vi "Receive Value Change Event.vi"(8 "error in (no error)":errorcluster, 10 "ValueChangeMsg":refnum<class "ValueChangeMsg.lvclass">, 11 "MediatorBusMonitor In":refnum<class "MediatorBusMonitor.lvclass">) -> (0 "error out":errorcluster, 3 "MediatorBusMonitor Out":refnum<class "MediatorBusMonitor.lvclass">)   [LabVIEW 2017, in "Mediator.lvlib" / "MediatorBusMonitor.lvclass"]
doc: "<License>\nCopyright © 2017 Composed Systems, LLC | All rights reserved\nwww.composed.io\n\nAuthor: Ethan Stern <ethan.stern@composed.io>\n\nThis software is provided \"AS IS\" WITHOUT WARRANTIES, either express or implied, AND IS FOR EDUCATIONAL PURPOSES ONLY.\n</License>"
uses:
  MediatorBusMonitor.lvclass
  ActorEvents/IEventAggregator Messages/ValueChangeMsg/ValueChangeMsg.lvclass
  ActorEvents/IEventAggregator Messages/ValueChangeMsg/ValueChangeMsg.lvclass/ValueChangeMsg.ctl
  MediatorBusMonitor.lvclass/MediatorBusMonitor.ctl
  gpm_packages/@cs/lookup-table/Source/LookupTable/LookupTable.lvclass/LookupTable.ctl
  gpm_packages/@cs/lookup-table/Source/LookupTable/Read Table Reference.vi
  gpm_packages/@cs/lookup-table/Source/LookupTable/LookupTable.lvclass
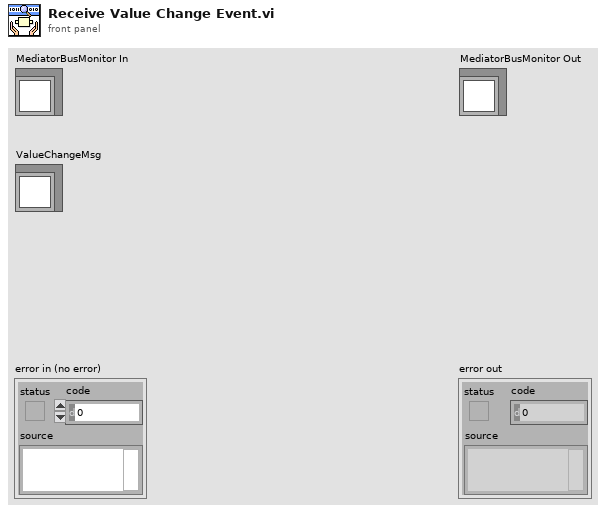
[diagram p1: front panel]
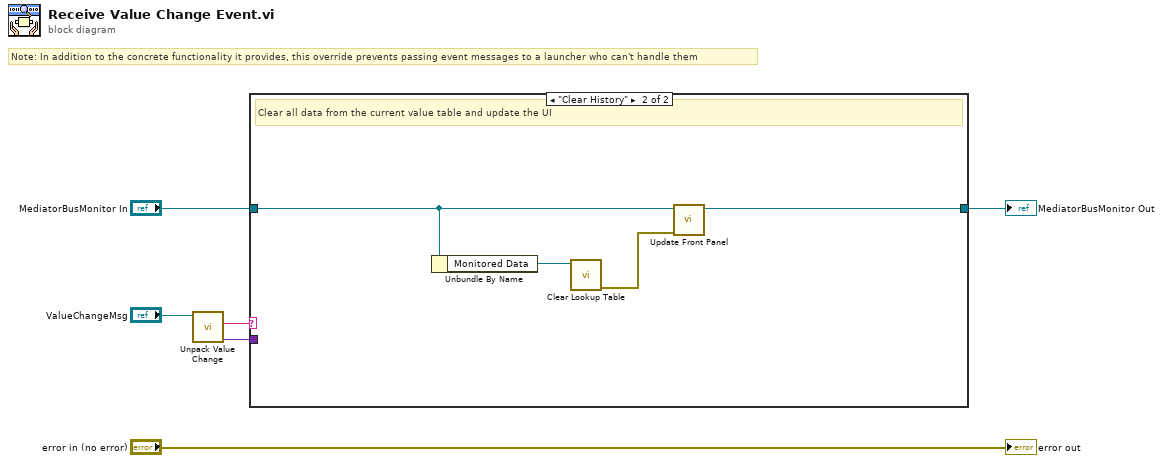
[diagram p0: block diagram]
diagram:
  # "Note: In addition to the concrete functionality it provides, this override prevents passing event messages to a launcher who can't handle them"
  n1 = call "Unpack Value Change.vi"("ValueChangeMsg"="ValueChangeMsg") -> ("New Value"=w2:variant, "Control Label"=w1:string)  [unwired: 6 in, 3 out]
  n2 = case shown="\"Clear History\"" w1 {
    tunnel: "MediatorBusMonitor In" -> [w7 w11]
    tunnel: [w7 w9] -> w3
    tunnel: w2 -> [_ _]
    frame Default {
      # "Do nothing by default -- And DO NOT relay anything to caller"
    }
    frame "Clear History" {
      # "Clear all data from the current value table and update the UI"
      n3 = Unbundle By Name(w11) -> ("Monitored Data"=w10:refnum<data-value>)
      n4 = call "Clear Lookup Table.vi"("LookupTable Reference"=w10) -> ("error out"=w8:errorcluster)  [unwired: 9 in, 1 out]
      n5 = call "Update Front Panel.vi"("error in (no error)"=w8, "MediatorBusMonitor In"=w11) -> ("MediatorBusMonitor Out"=w9:refnum<class "MediatorBusMonitor.lvclass">)  [unwired: 8 in, 1 out]
    }
  }
  "MediatorBusMonitor Out" <- w3
  "error out" <- "error in (no error)"
